vi "光照强度历史数据.vi"(10 "亮度显示":dbl, 11 "移位输入":string[][](array[string])) -> (3 "移位输出":string[][](array[string]))   [LabVIEW 2016]
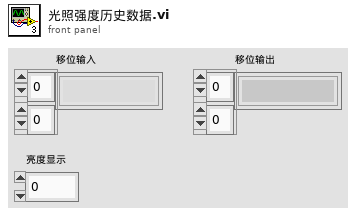
[diagram p1: front panel]
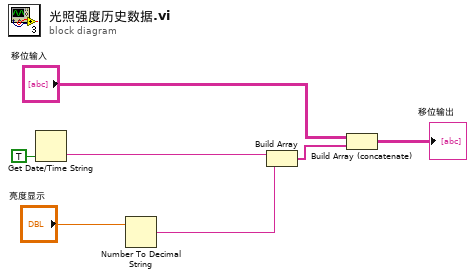
[diagram p0: block diagram]
diagram:
  n1 = Get Date/Time String(want seconds? (F)=TRUE ("需要秒？(F)")) -> (time string=w6:string)  [unwired: 2 in, 1 out]
  n2 = Number To Decimal String(number="亮度显示") -> (decimal integer string=w4:string)  [unwired: 1 in]
  n3 = Build Array(w6, w4) -> (w7:string[])
  n4 = Build Array (concatenate)("移位输入", w7) -> (→"移位输出":string[][])
